vi "MARELE.vi"() -> ()   [LabVIEW 2015]
uses:
  C:/Users/MAHA/Desktop/delele/bin/Debug/delele.dll
panel:
  out "output 2":i32
  out "output 1":i32
  in  "Path 7":path
  out "return type":i32
  in  "Path 6":path
  in  "Path 5":path
  in  "Path 4":path
  in  "Path 3":path
  in  "Path 2":path
  in  "Path":path
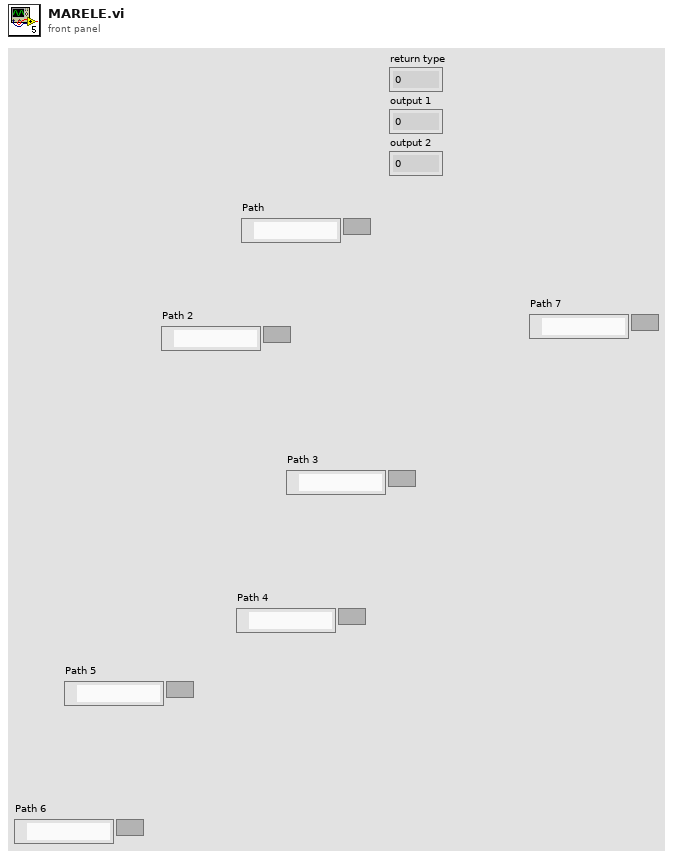
[diagram p1: front panel]
types:
  T1 = enum16{"open", "replace", "create", "open or create", "replace or create", "replace or create with confirmation"}
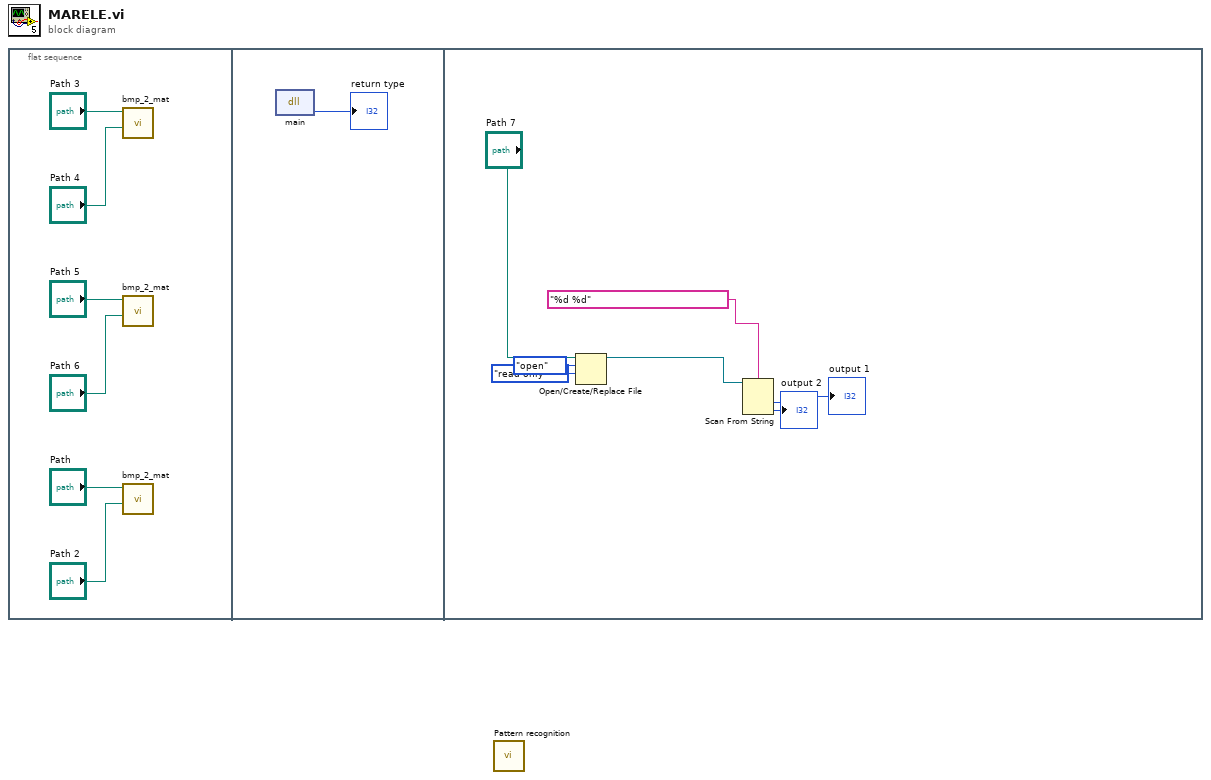
[diagram p0: block diagram]
diagram:
  n1 = flat-sequence {
    frame #0 {
      n2 = call "bmp_2_mat.vi"("Destinatia1"="Path 4", "Imaginea1"="Path 3") -> ()  [unwired: 10 in]
      n3 = call "bmp_2_mat.vi"("Destinatia1"="Path 6", "Imaginea1"="Path 5") -> ()  [unwired: 10 in]
      n4 = call "bmp_2_mat.vi"("Destinatia1"="Path 2", "Imaginea1"="Path") -> ()  [unwired: 10 in]
    }
    frame #1 {
      n5 = dll-call lib="C:/Users/MAHA/Desktop/delele/bin/Debug/delele.dll" fn="main"() -> ("return type"=→"return type":i32)  [unwired: 3 in, 2 out]
    }
    frame #2 {
      n6 = Open/Create/Replace File(file path (use dialog)="Path 7", operation (0:open)=T1."open", access (0:read/write)=enum16{"read/write", "read-only", "write-only"}."read-only") -> (refnum out=w11:refnum<file>)  [unwired: 3 in, 2 out]
      n7 = Scan From String("%d %d" ("format string"), w11) -> (output 1=→"output 1":i32, output 2=→"output 2":i32)  [unwired: 3 in, 2 out]
    }
  }
  n8 = call "Pattern recognition.vi"() -> ()  [unwired: 12 in]
